vi "TLPM Initialize2.vi"(8 "error in (no error)":errorcluster {"code" format="%.0x"}, 9 "Reset Device (Reset Device)":bool=TRUE, 10 "ID Query (Do Query)":bool=TRUE, 11 "resource name":refnum<visa-resource-name>) -> (0 "error out":errorcluster {"code" format="%.0x"}, 3 "instrument handle out":refnum<visa-resource-name>)   [LabVIEW 2023, in "Thorlabs Power Meter.lvlib"]
doc: "This VI initializes the instrument driver session and performs the following initialization actions:\n\n(1) Opens a session to the Default Resource Manager resource and a session to the specified device using the Resource Name.\n(2) Performs an identification query on the instrument.\n(3) Resets the instrument to a known state.\n(4) Sends initialization commands to the instrument.\n(5) Returns an instrument handle which is used to distinguish between different sessions of this instrument driver.\n\nNotes:\n(1) Each time this VI is invoked a unique session is opened."
uses:
  Thorlabs Power Meter.lvlib
panel:
  # "(C) 2021 National Instruments.  ALL RIGHTS RESERVED."
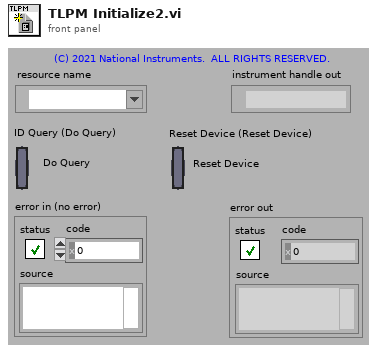
[diagram p1: front panel]
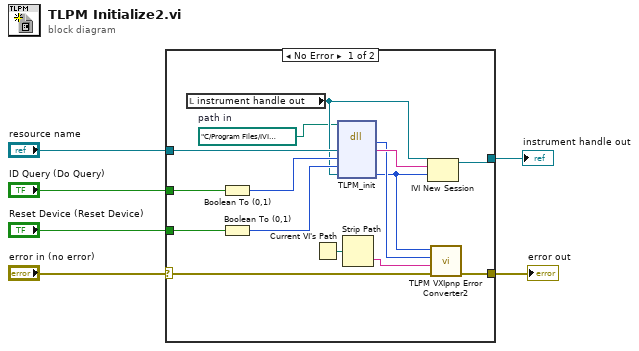
[diagram p0: block diagram]
diagram:
  n1 = case shown="No Error" "error in (no error)" {
    selector: "error in (no error)" -> [w11 w22]
    tunnel: [w12 w22] -> w5
    tunnel: "resource name" -> [w17 _]
    tunnel: [w16 _] -> w3
    tunnel: "ID Query (Do Query)" -> [w14 _]
    tunnel: "Reset Device (Reset Device)" -> [w13 _]
    frame No Error {
      w7 = path "C:/Program Files/IVI Foundation/VISA/Win64/Bin/TLPM_64.dll"  # path in
      n2 = local read "instrument handle out"() -> (w15:refnum<visa-resource-name>)
      n3 = Boolean To (0,1)(Boolean=w14) -> (0, 1=w21:i16)
      n4 = Boolean To (0,1)(Boolean=w13) -> (0, 1=w20:i16)
      n5 = Current VI's Path() -> (path=w18:path)
      n6 = dll-call lib="TLPM_64.dll" fn="TLPM_init"(path in=w7, "resource name"=w17, "id query"=w21, "reset device"=w20, "instrument handle"=w15) -> ("status"=w9:i32, "resource name"=w19:string, "instrument handle"=w8:u32)  [unwired: 4 in, 2 out]
      n7 = Strip Path(path=w18) -> (name=w10:string)  [unwired: 1 out]
      n8 = IVI New Session(9:w8, 10:w19, 11:w15) -> (3:w16:refnum<visa-resource-name>)
      n9 = call "TLPM VXIpnp Error Converter2.vi"("error in (no error)"=w11, "Name Of VI (\"\")"=w10, "CVI Error Code (0)"=w9, "instrument handle"=w8) -> ("error out"=w12:errorcluster)  [unwired: 6 in, 1 out]
    }
    frame Error {
    }
  }
  "error out" <- w5
  "instrument handle out" <- w3
